vi "Trapi162FXP.vi"(9 "N El. to Ave.":i32, 11 "Trap Data":i16[](array[numeric])) -> (1 "Trap 2":fxp<+/-,16,1>, 3 "Trap 1":fxp<+/-,16,1>)   [LabVIEW 2013]
uses:
  <vilib>/Analysis/baseanly.llb/Mean (DBL).vi
  <vilib>/Analysis/NI_AALBase.lvlib
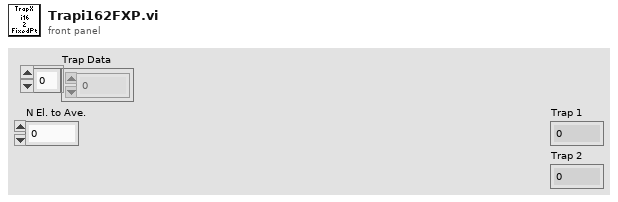
[diagram p1: front panel]
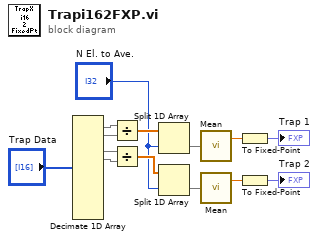
[diagram p0: block diagram]
diagram:
  n1 = Decimate 1D Array("Trap Data") -> (w8:i16[], w9:i16[], w11:i16[], w12:i16[])  [unwired: 9 out]
  n2 = Divide(x=w8, y=w9) -> (x/y=w7:dbl[])
  n3 = Divide(x=w11, y=w12) -> (x/y=w10:dbl[])
  n4 = Split 1D Array(array=w7, index="N El. to Ave.") -> (second subarray=w5:dbl[])  [unwired: 1 out]
  n5 = Split 1D Array(array=w10, index="N El. to Ave.") -> (second subarray=w6:dbl[])  [unwired: 1 out]
  n6 = call-poly <vilib>:"Mean.vi"("X"=w5) -> ("mean"=w13:dbl)  [unwired: 1 out]
  n7 = call-poly <vilib>:"Mean.vi"("X"=w6) -> ("mean"=w14:dbl)  [unwired: 1 out]
  n8 = To Fixed-Point(number=w13) -> (fixed-point=→"Trap 1":fxp<+/-,16,1>)  [unwired: 1 in]
  n9 = To Fixed-Point(number=w14) -> (fixed-point=→"Trap 2":fxp<+/-,16,1>)  [unwired: 1 in]
